vi "ItemByName.vi"(7 "LabVIEW Object Type":refnum<class>, 8 "error in (no error)":errorcluster, 10 "Name":string, 11 "Collection in":refnum<class "CollectionByValue.lvclass">) -> (0 "error out":errorcluster, 1 "found":bool, 2 "LabVIEW Object":refnum<class>, 3 "Collection out":refnum<class "CollectionByValue.lvclass">)   [LabVIEW 2021, in "Collection.lvlib" / "CollectionByValue.lvclass"]
uses:
  CollectionByValue.lvclass
  CollectionByValue.lvclass/CollectionByValue.ctl
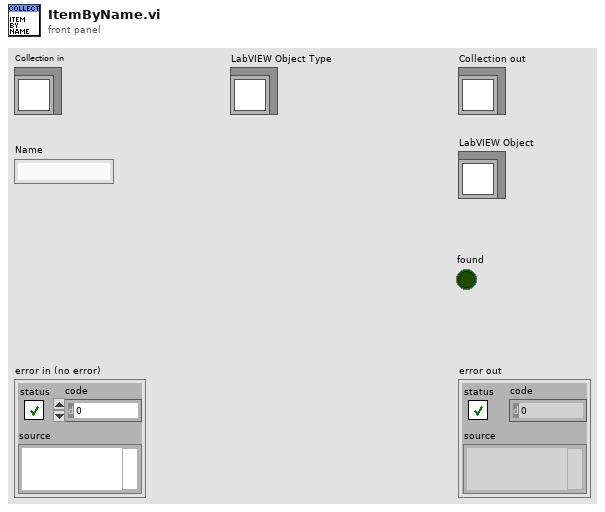
[diagram p1: front panel]
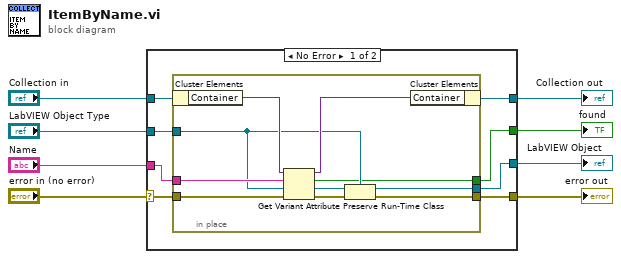
[diagram p0: block diagram]
diagram:
  n1 = case shown="No Error" "error in (no error)" {
    selector: "error in (no error)" -> [w16 w29]
    tunnel: [w15 w29] -> w7
    tunnel: [w13 w28] -> w5
    tunnel: "Collection in" -> [w14 w28]
    tunnel: "Name" -> [w12 _]
    tunnel: "LabVIEW Object Type" -> [w11 w27]
    tunnel: [w10 w27] -> w2
    tunnel: [w9 _] -> w1
    frame No Error {
      n2 = in-place {
        in-place-border: w16 -> [w26]
        in-place-border: [w21] -> w15
        in-place-border: w12 -> [w23]
        in-place-border: w11 -> [w19]
        in-place-border: [w18] -> w10
        in-place-border: [w17] -> w9
        n3 = in-place-cluster #1(w14) -> ("Container"=w25:variant)
        n4 = Get Variant Attribute(Variant=w25, name=w23, default value (empty Variant)=w19, error in=w26) -> (duplicate Variant=w24:variant, found=w17:bool, value=w20:refnum<class>, error out=w22:errorcluster)
        n5 = Preserve Run-Time Class(object in=w20, error in=w22, 2:w19) -> (object out=w18:refnum<class>, error out=w21:errorcluster)
        n6 = in-place-cluster #1("Container"=w24) -> (w13:refnum<class "CollectionByValue.lvclass">)
      }
    }
    frame Error {
    }
  }
  "error out" <- w7
  "Collection out" <- w5
  "LabVIEW Object" <- w2
  "found" <- w1
